vi "saveZstack.vi"(0 "z-stack_in":dbl[][][](array[numeric]), 1 "image-step_size":dbl=0.025, 2 "image-dwell_time":dbl=0.01 format="%.3f", 5 "image_start_xyz":T2 {"Z start" format="%#.4g"; "Y start" format="%#.4g"; "X start" format="%#.4g"}, 7 "image_size_xy":cluster{"X image size":dbl, "Y image size":dbl}={"X image size"=1.25, "Y image size"=1.25}, 9 "micro_pos-xyz":T1, 11 "tile_n_xy":cluster{"tile_n_x":i32, "tile_n_y":i32}={"tile_n_x"=1, "tile_n_y"=1}, 13 "Objective":string="objective01") -> ()   [LabVIEW 2014]
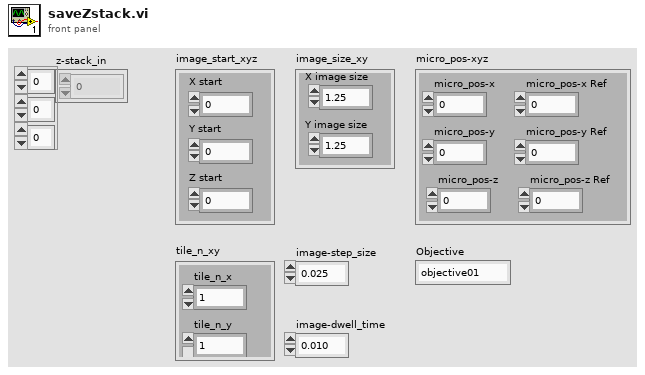
[diagram p1: front panel]
types:
  T1 = cluster{"micro_pos-x":dbl, "micro_pos-y":dbl, "micro_pos-z":dbl, "micro_pos-x Ref":dbl, "micro_pos-y Ref":dbl, "micro_pos-z Ref":dbl}
  T2 = cluster{"X start":dbl, "Y start":dbl, "Z start":dbl}
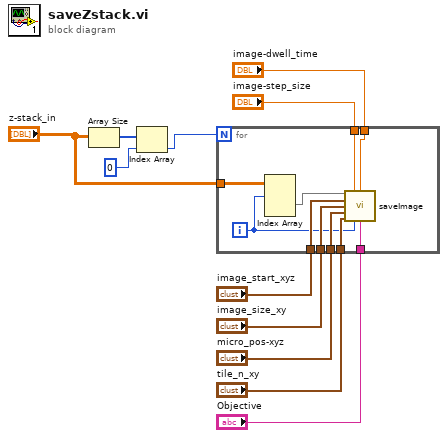
[diagram p0: block diagram]
diagram:
  n1 = Array Size(array="z-stack_in") -> (size(s)=w8:i32[])
  n2 = Index Array(array=w8, index=0) -> (element=w10:i32)
  n3 = for {
    N: w10 -> [_]
    tunnel: "z-stack_in" -> [w21]
    tunnel: "image-step_size" -> [w19]
    tunnel: "image-dwell_time" -> [w18]
    tunnel: "image_start_xyz" -> [w17]
    tunnel: "image_size_xy" -> [w16]
    tunnel: "micro_pos-xyz" -> [w15]
    tunnel: "tile_n_xy" -> [w14]
    tunnel: "Objective" -> [w12]
    i -> [w13]
    n4 = Index Array(array=w21, index (dim 0)=w13) -> (element=w20:dbl[][])  [unwired: 2 in]
    n5 = call "saveImage.vi"("image"=w20, "image-step_size"=w19, "image-dwell_time"=w18, "image_start_xyz"=w17, "image_size_xy"=w16, "micro_pos-xyz"=w15, "tile_n_xy"=w14, "run_number"=w13, "Objective"=w12) -> ()  [unwired: 6 in, 1 out]
  }
